vi "TheGoodStuff.vi"() -> ()   [LabVIEW 2021]
panel:
  in  "Please click me <3":bool
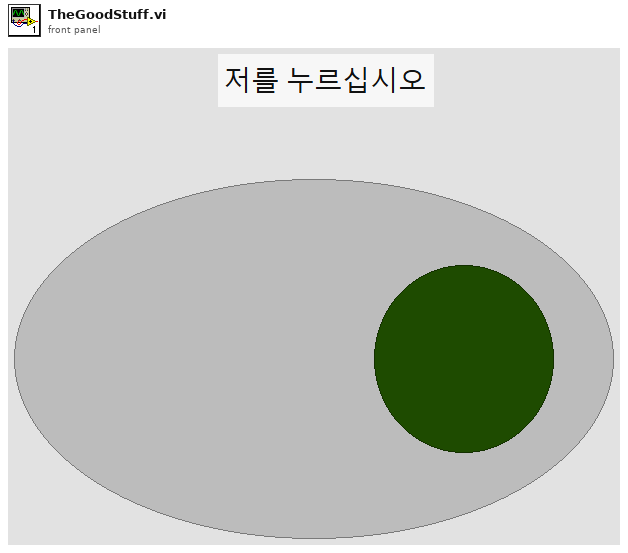
[diagram p1: front panel]
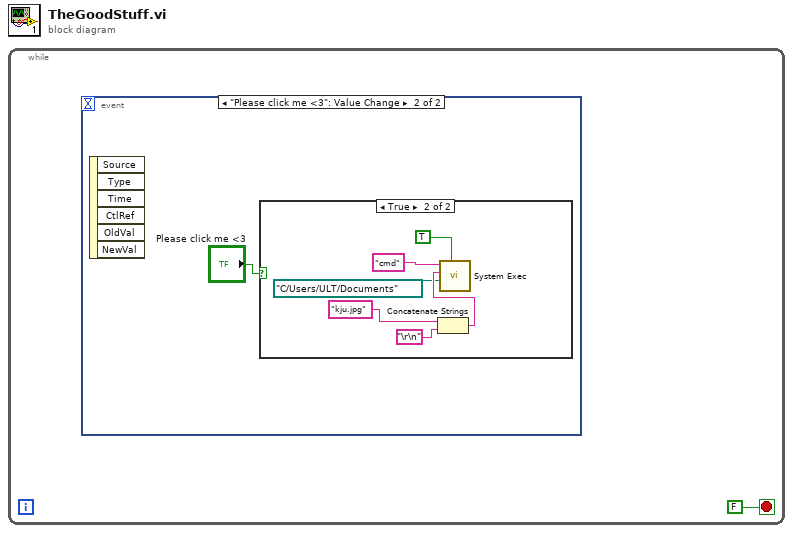
[diagram p0: block diagram]
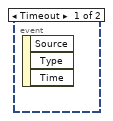
[diagram p2: hidden frame]
diagram:
  n1 = while {
    stop <- FALSE stop-if-true
    n2 = event shown="[1] \"Please click me <3\": Value Change" {
      selector: _ -> [_ _]
      dyn-events: _ -> [_ _]
      timeout: _ -> [_ _]
      event Timeout {
        n3 = event-data() -> ()  [unwired: 1 in, 3 out]
      }
      event "Please click me <3": Value Change {
        n4 = event-data() -> ()  [unwired: 1 in, 6 out]
        n5 = case shown="True" "Please click me <3" {
          frame False {
          }
          frame True {
            n6 = Concatenate Strings("kju.jpg" ("standard input"), "\r\n") -> (w5:string)
            n7 = call <vilib>:"System Exec.vi"("wait until completion? (T)"=TRUE, "working directory"=path "C:/Users/ULT/Documents", "standard input"=w5, "command line"="cmd") -> ()  [unwired: 4 in, 4 out]
          }
        }
      }
    }
  }
